vi "File.Get Relative Path.vi"(8 "error in":errorcluster, 10 "Root Dir":path, 11 "Path":path) -> (0 "error out":errorcluster, 3 "Relative Path":string)   [LabVIEW 2018]
uses:
  Errors/Error.Error Code List.ctl
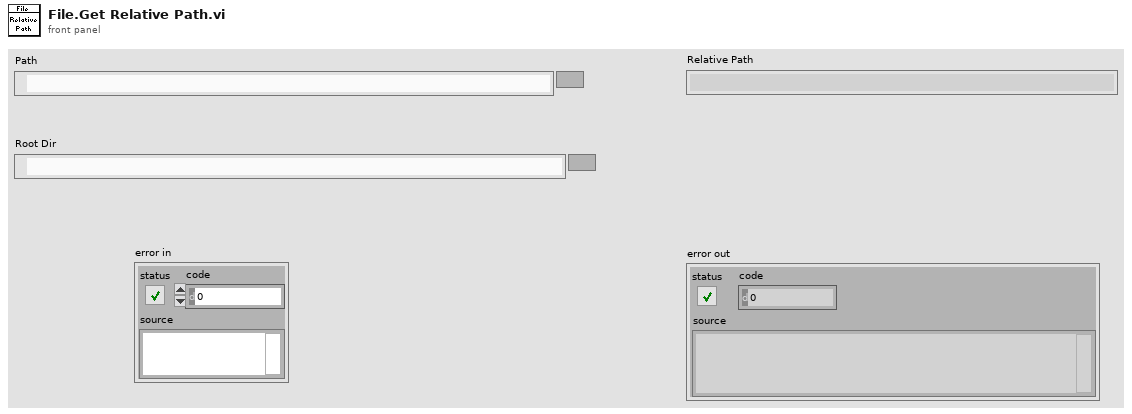
[diagram p1: front panel]
types:
  T1 = typedef "Error.Error Code List.ctl" = i32
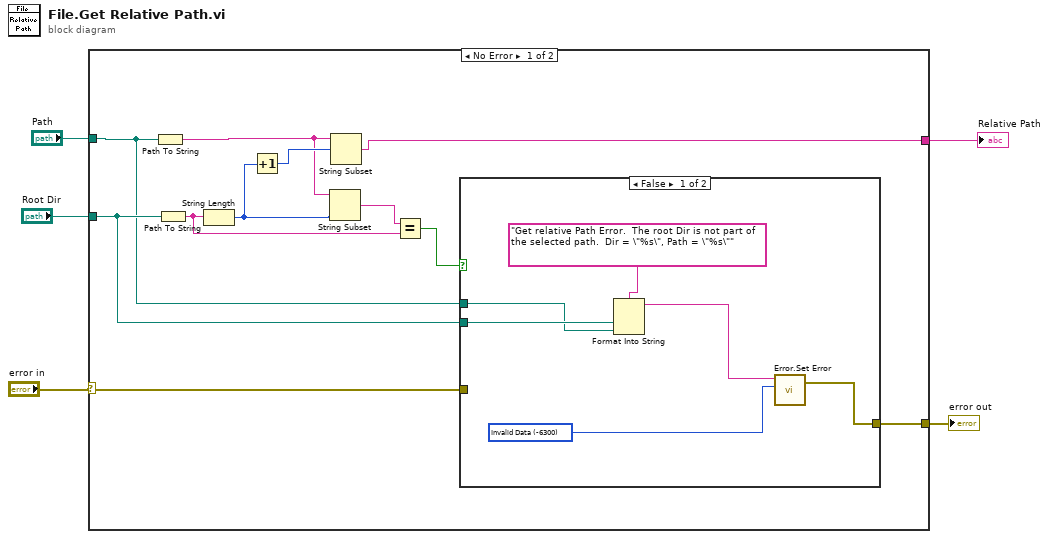
[diagram p0: block diagram]
diagram:
  n1 = case shown="No Error" "error in" {
    selector: "error in" -> [w9 w23]
    tunnel: "Root Dir" -> [w7 _]
    tunnel: "Path" -> [w6 _]
    tunnel: [w10 _] -> w3
    tunnel: [w8 w23] -> w1
    frame No Error {
      n2 = Path To String(path=w6) -> (string=w15:string)
      n3 = Path To String(path=w7) -> (string=w12:string)
      n4 = String Length(string=w12) -> (length=w14:i32)
      n5 = Increment(x=w14) -> (x+1=w16:i32)
      n6 = String Subset(string=w15, length (rest)=w14) -> (substring=w13:string)  [unwired: 1 in]
      n7 = String Subset(string=w15, offset (0)=w16) -> (substring=w10:string)  [unwired: 1 in]
      n8 = Equal?(x=w13, y=w12) -> (x = y?=w11:bool)
      n9 = case shown="False" w11 {
        tunnel: w9 -> [_ _]
        tunnel: [w19 _] -> w8
        tunnel: w7 -> [w18 _]
        tunnel: w6 -> [w17 _]
        frame False {
          w22 = T1 -6300 items=["No Error"=0, "Abort"=-2, "Misc"=-5000, "Fixture Error"=-5100, "File IO - General"=-5200, "FIle IO - Config Error"=-5201, "Instrument - General"=-5300, "Instrument - Serial Com"=-5301, "Instrument - Camera"=-5302, "Instrument - PS"=-5303, "Instrument - Oscilloscope"=-5304, "Instrument - Function Gen"=-5305, "Instrument - Load"=-5306, "Instrument - Meter"=-5307, "Instrument - Power Control"=-5308, "Instrument - Motion"=-5309, "Instrument - RF"=-5310, "System Exe"=-5400, "Image Processing"=-5500, "Communication"=-5600, "Script - Syntax Error"=-6000, "Script - Invalid Name or Param"=-6100, "Script - Timeout"=-6200, "Invalid Data"=-6300, "FW Update Error"=-6500] ("Std Code")
          n10 = Format Into String(format string="Get relative Path Error.  The root Dir is not part of the selected path.  Dir = \"%s\", Path = \"%s\"" ("Desc"), w18, w17) -> (resulting string=w20:string)  [unwired: 2 in, 1 out]
          n11 = call "Error.Set Error.vi"("Code"=w22, "Desc"=w20) -> ("error out"=w19:errorcluster)  [unwired: 5 in]
        }
        frame True {
        }
      }
    }
    frame Error {
    }
  }
  "error out" <- w1
  "Relative Path" <- w3
